vi "ini_object_parse_array.vi"(8 "error in":errorcluster, 11 "variant in":variant) -> (0 "error out":errorcluster, 1 "dims":i16, 2 "error":string, 3 "type id":i16)   [LabVIEW 2018]
panel:
  out "type string":i16[](array[numeric]) format="%04x"
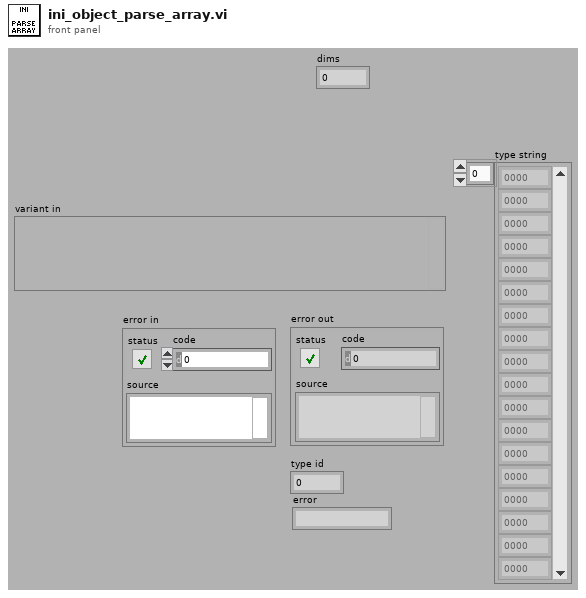
[diagram p1: front panel]
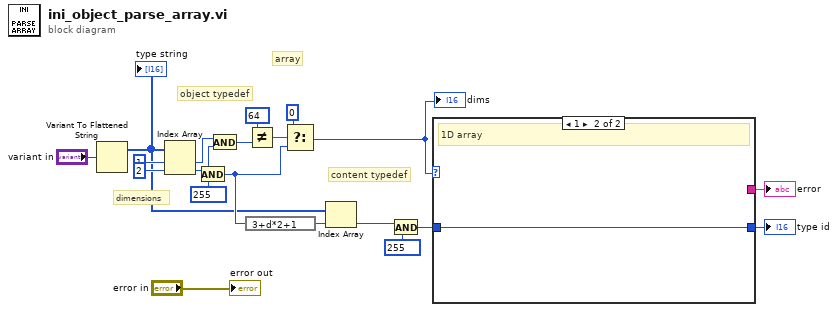
[diagram p0: block diagram]
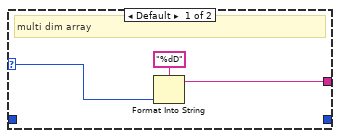
[diagram p2: hidden frame]
diagram:
  w10 = i16 255 ("y")
  # "content typedef"
  # "dimensions"
  # "array"
  # "object typedef"
  n1 = Variant To Flattened String(Variant="variant in") -> (1:w3:i16[])  [unwired: 1 out]
  "type string" <- w3
  n2 = Index Array(array=w3, index #1=1 ("index"), index #2=2 ("index")) -> (element #1=w11:i16, element #2=w18:i16)
  n3 = And(x=w18, y=w10) -> (x .and. y?=w4:i16)
  n4 = And(x=w11, y=w10) -> (x .and. y?=w9:i16)
  n5 = expression code="3+d*2+1"(w4) -> (w2:i16)
  n6 = Not Equal?(x=i16 64, y=w9) -> (x != y?=w7:bool)
  n7 = Select(t=i16 0, s=w7, f=w4) -> (s? t:f=w6:i16)
  "dims" <- w6
  n8 = Index Array(array=w3, index=w2) -> (element=w1:i16)
  n9 = And(x=w1, y=i16 255) -> (x .and. y?=w16:i16)
  n10 = case shown="1" w6 {
    selector: w6 -> [w22 _]
    tunnel: w16 -> [_ w24]
    tunnel: [_ w24] -> w15
    tunnel: [w21 _] -> w14
    frame Default {
      # "multi dim array"
      n11 = Format Into String(format string="%dD", w22) -> (resulting string=w21:string)  [unwired: 2 in, 1 out]
    }
    frame 1 {
      # "1D array"
    }
  }
  "type id" <- w15
  "error" <- w14
  "error out" <- "error in"
